vi "p1.vi"() -> ()   [LabVIEW 2025, in "d9.lvlib"]
uses:
  d9.lvlib
  16714bf5-c3b5-47bb-b419-980da8f6e6cb.vi
  <vilib>/Comparison/Less/Less Functor/Less Functor.lvclass
  AOC/AOC.lvlib
panel:
  out "red tile 2":T1
  out "red tile 1":T1
  out "Floor Plan":T2(graph)
  out "Area":u64
  in  "Example":string="7,1\n11,1\n11,7\n9,7\n9,5\n2,5\n2,3\n7,3"
  in  "Example":bool
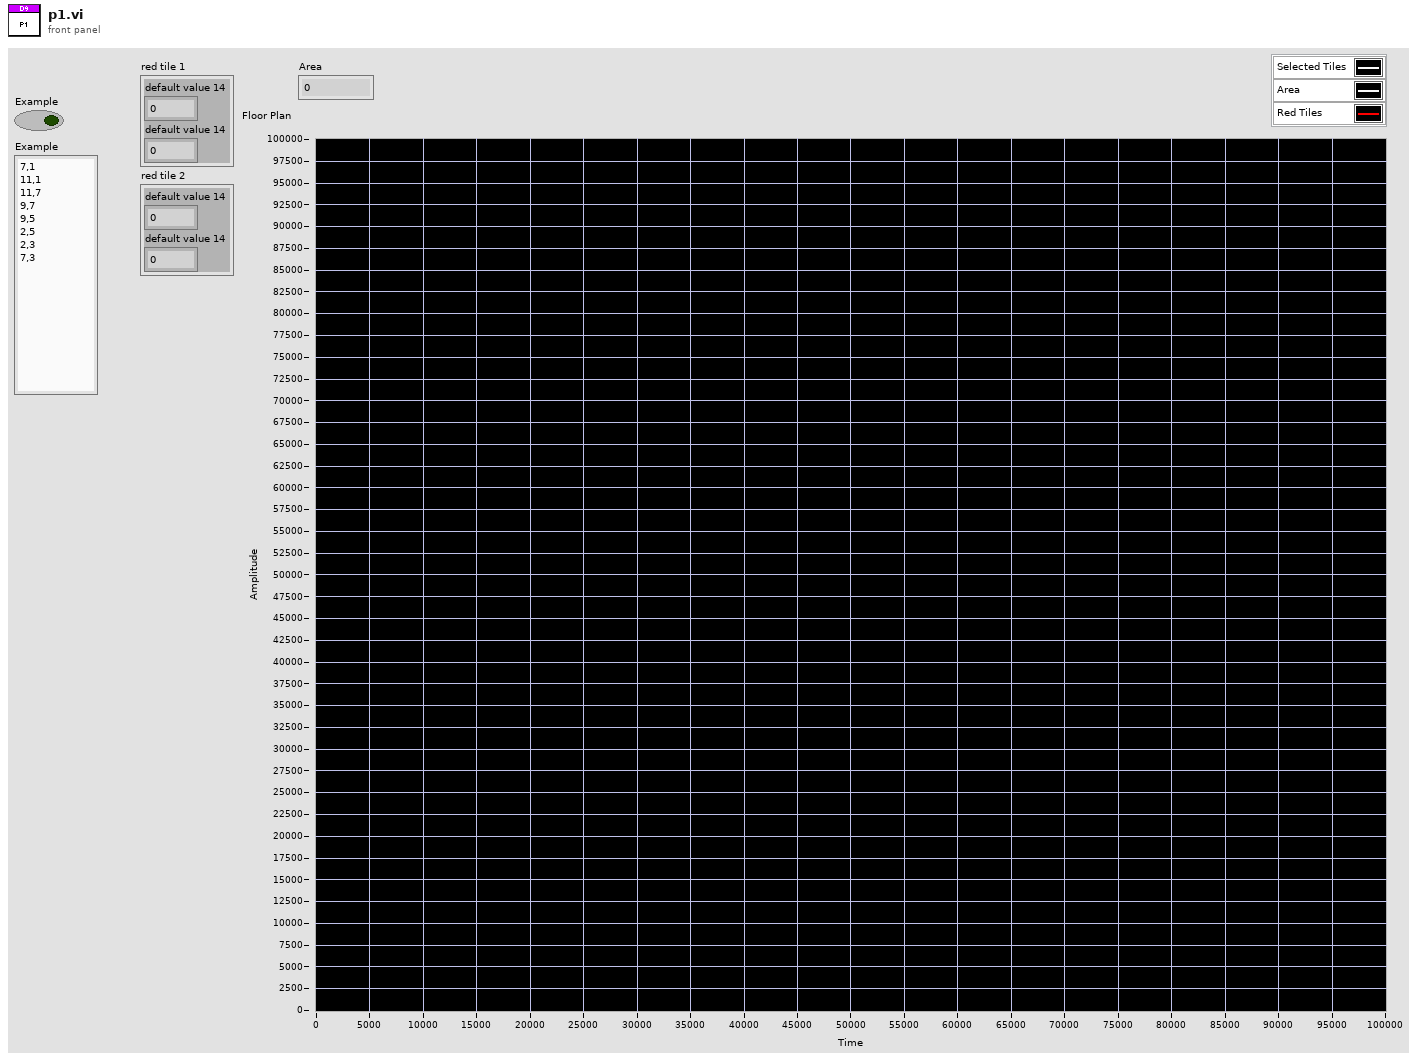
[diagram p1: front panel]
types:
  T1 = cluster{"default value 14":i64, "default value 14":i64}
  T2 = cluster{cluster{"default value 14":i64, "default value 14":i64}[]}[]
  T3 = cluster{"default value 14":i64, "default value 14":i64}[]
  T4 = cluster{cluster{"default value 14":i64, "default value 14":i64}[]}
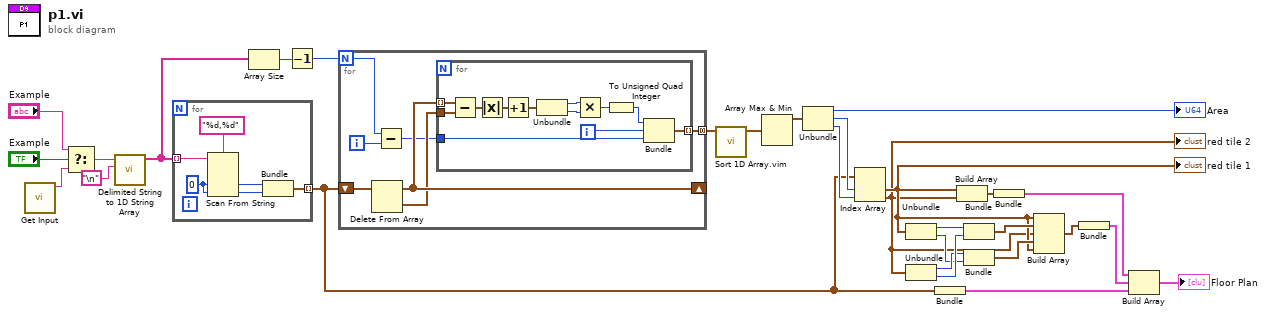
[diagram p0: block diagram]
diagram:
  n1 = call "Get Input.vi"() -> ("Input"=w27:string)  [unwired: 11 in]
  n2 = Select(t="Example", s="Example", f=w27) -> (s? t:f=w1:string)
  n3 = call <vilib>:"Delimited String to 1D String Array.vi"("delimiter"="\n", "delimited string"=w1) -> ("string array"=w25:string[])  [unwired: 9 in]
  n4 = for {
    tunnel: w25 -> [w35] mode=indexing
    tunnel: [w31] -> w16 mode=indexing
    w30 = i64 0 ("default value 14")
    n5 = Scan From String(format string="%d,%d", input string=w35, default 1=w30, default 2=w30) -> (output 1=w33:i64, output 2=w32:i64)  [unwired: 2 in, 3 out]
    n6 = Bundle("default value 14"=w33, "default value 14"=w32) -> (w31:T1)  [unwired: 1 in]
  }
  n7 = Array Size(array=w25) -> (size(s)=w24:i32)
  n8 = Decrement(x=w24) -> (x-1=w23:i32)
  n9 = for {
    N: w23 -> [w36]
    shift-right: [w41] -> _
    shift-left: w16 -> [w42]
    tunnel: [w39] -> w19 mode=concatenating
    i -> [w37]
    n10 = Delete From Array(array=w42) -> (deleted portion=w40:T1, array with subset deleted=w41:T3)  [unwired: 2 in]
    n11 = Subtract(x=w36, y=w37) -> (x-y=w38:i32)
    n12 = for {
      tunnel: w41 -> [w54] mode=indexing
      tunnel: w40 -> [w53]
      tunnel: w38 -> [w46]
      tunnel: [w45] -> w39 mode=indexing
      i -> [w47]
      n13 = Subtract(x=w54, y=w53) -> (x-y=w52:T1)
      n14 = Absolute Value(x=w52) -> (abs(x)=w51:T1)
      n15 = Increment(x=w51) -> (x+1=w43:T1)
      n16 = Unbundle(w43) -> ("default value 14"=w50:i64, "default value 14"=w49:i64)
      n17 = Multiply(x=w50, y=w49) -> (x*y=w48:i64)
      n18 = To Unsigned Quad Integer(1:w48) -> (0:w44:u64)
      n19 = Bundle(w44, w47, w46) -> (w45:cluster{u64, i32, i32})  [unwired: 1 in]
    }
  }
  n20 = call "Sort 1D Array.vim"("unsorted array"=w19) -> ("sorted array"=w18:cluster{u64, i32, i32}[])  [unwired: 10 in]
  n21 = Array Max & Min(array=w18) -> (max value=w22:cluster{u64, i32, i32})  [unwired: 3 out]
  n22 = Unbundle(w22) -> (→"Area":u64, w21:i32, w17:i32)
  n23 = Index Array(array=w16, index #1=w21, index #2=w17) -> (element #1=w3:T1, element #2=w2:T1)
  "red tile 1" <- w3
  "red tile 2" <- w2
  n24 = Unbundle(w3) -> ("default value 14"=w11:i64, "default value 14"=w5:i64)
  n25 = Unbundle(w2) -> ("default value 14"=w6:i64, "default value 14"=w10:i64)
  n26 = Bundle(w16) -> (w15:T4)  [unwired: 1 in]
  n27 = Build Array(w3, w2) -> (w13:T3)
  n28 = Bundle("default value 14"=w11, "default value 14"=w10) -> (w9:T1)  [unwired: 1 in]
  n29 = Bundle("default value 14"=w6, "default value 14"=w5) -> (w4:T1)  [unwired: 1 in]
  n30 = Bundle(w13) -> (w12:T4)  [unwired: 1 in]
  n31 = Build Array(w3, w9, w2, w4, w3) -> (w7:T3)
  n32 = Bundle(w7) -> (w8:T4)  [unwired: 1 in]
  n33 = Build Array(w12, w8, w15) -> (→"Floor Plan":T2)
